vi "ConstellationClose.vi"(8 "error in":errorcluster, 11 "Task out":refnum<visa-resource-name>[](array[refnum])=["COM8"]) -> (0 "error out":errorcluster)   [LabVIEW 2012]
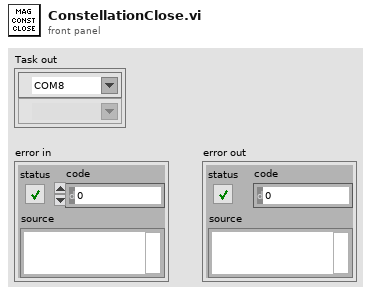
[diagram p1: front panel]
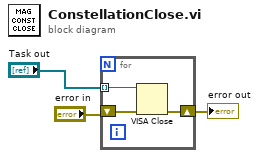
[diagram p0: block diagram]
diagram:
  n1 = for {
    tunnel: "Task out" -> [w6] mode=indexing
    shift-right: [w4] -> w1
    shift-left: "error in" -> [w5]
    n2 = VISA Close(VISA resource name=w6, error in (no error)=w5) -> (error out=w4:errorcluster)
  }
  "error out" <- w1
